vi "Write File-group-channel.vi"(8 "error in (no error)":errorcluster, 10 "File-group-channel":T1(array[cluster]), 11 "XY Plot in":refnum<class "XY Plot.lvclass">) -> (0 "error out":errorcluster, 3 "XY Plot out":refnum<class "XY Plot.lvclass">)   [LabVIEW 2015, in "XY Plot.lvclass"]
uses:
  XY Plot.lvclass
  XY Plot.lvclass/XY Plot.ctl
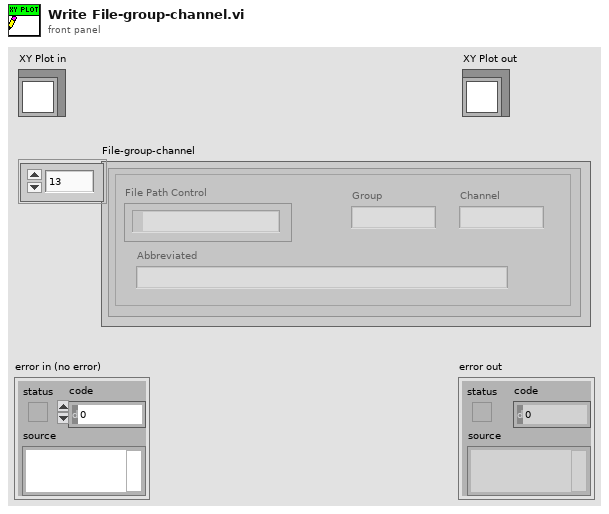
[diagram p1: front panel]
types:
  T1 = cluster{"File Path Control":path, "Group":string, "Channel":string, "Abbreviated":string}[]
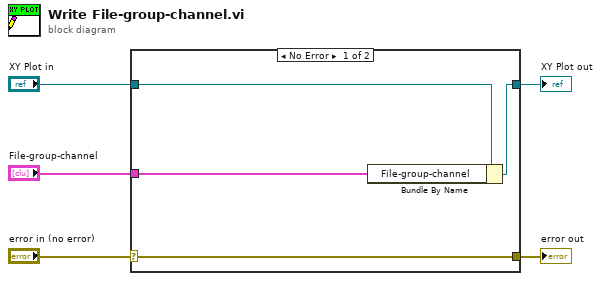
[diagram p0: block diagram]
diagram:
  n1 = case shown="No Error" "error in (no error)" {
    selector: "error in (no error)" -> [w9 w10]
    tunnel: [w9 w10] -> w4
    tunnel: [w7 w11] -> w2
    tunnel: "XY Plot in" -> [w8 w11]
    tunnel: "File-group-channel" -> [w6 _]
    frame No Error {
      n2 = Bundle By Name(cluster=w8, "File-group-channel"=w6) -> (w7:refnum<class "XY Plot.lvclass">)
    }
    frame Error {
    }
  }
  "error out" <- w4
  "XY Plot out" <- w2
